vi "Climb Logic Core.vi"(11 "Climb Controls":T2) -> (3 "Climb Outputs":T1, 5 "Climbing Override":bool)   [LabVIEW 2017]
uses:
  Climb Controls.ctl
  Climb Outputs.ctl
  Robot Global Data.vi
panel:
  in  "Hook Deploy":bool
  in  "Ramp Tail":bool
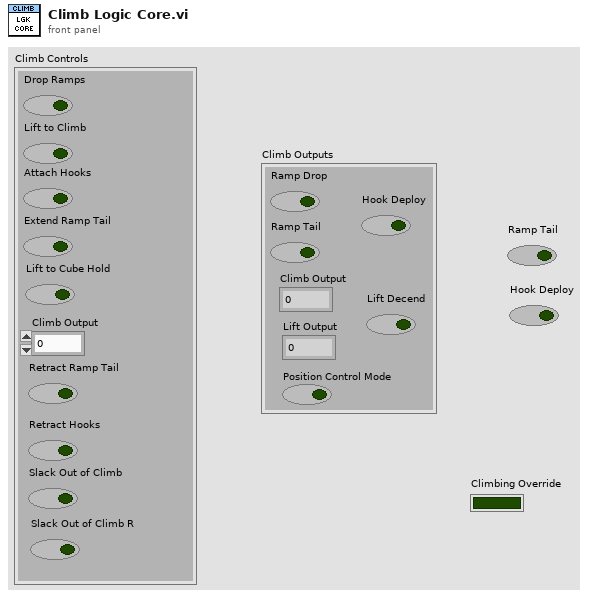
[diagram p1: front panel]
types:
  T1 = typedef "Climb Outputs.ctl" = cluster{"Ramp Drop":bool, "Ramp Tail":bool, "Climb Output":dbl, "Lift Output":dbl, "Position Control Mode":bool, "Hook Deploy":bool, "Lift Decend":bool}
  T2 = typedef "Climb Controls.ctl" = cluster{"Drop Ramps":bool, "Lift to Climb":bool, "Attach Hooks":bool, "Extend Ramp Tail":bool, "Climb Output":dbl, "Lift to Cube Hold":bool, "Retract Ramp Tail":bool, "Retract Hooks":bool, "Slack Out of Climb":bool, "Slack Out of Climb R":bool}
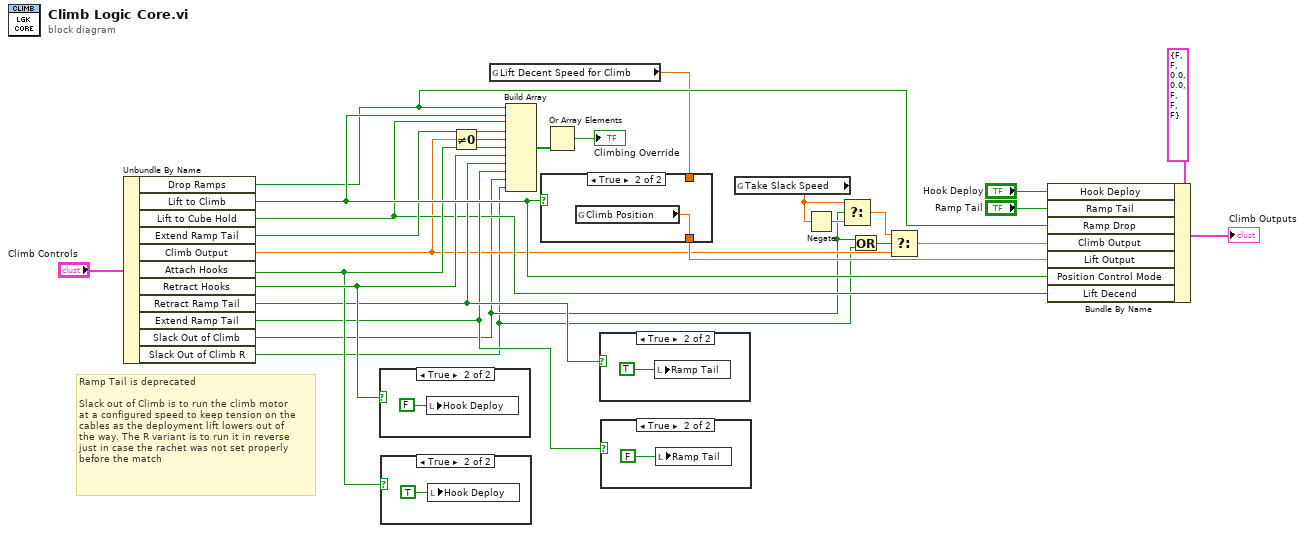
[diagram p0: block diagram]
diagram:
  # "Ramp Tail is deprecated\n\nSlack out of Climb is to run the climb motor\nat a configured speed to keep tension on the\ncables as the deployment lift lowers out of\nthe way. The R variant is to run it in reverse\njust in case the rachet was not set properly\nbefore the match"
  n1 = Unbundle By Name("Climb Controls") -> ("Drop Ramps"=w17:bool, "Lift to Climb"=w21:bool, "Lift to Cube Hold"=w9:bool, "Extend Ramp Tail"=w19:bool, "Climb Output"=w4:dbl, "Attach Hooks"=w14:bool, "Retract Hooks"=w15:bool, "Retract Ramp Tail"=w13:bool, "Extend Ramp Tail"=w12:bool, "Slack Out of Climb"=w2:bool, "Slack Out of Climb R"=w1:bool)
  n2 = case shown="True" w15 {
    frame False {
    }
    frame True {
      n3 = local write "Hook Deploy"(FALSE) -> ()
    }
  }
  n4 = case shown="True" w14 {
    frame False {
    }
    frame True {
      n5 = local write "Hook Deploy"(TRUE) -> ()
    }
  }
  n6 = Not Equal To 0?(x=w4) -> (x != 0?=w22:bool)
  n7 = global read "Robot Global Data.vi" "Lift Decent Speed for Climb"() -> (w10:dbl)
  n8 = Build Array(w17, w21, w9, w19, w22, w14, w15, w13, w12, w2, w1) -> (w24:bool[])
  n9 = case shown="True" w21 {
    tunnel: [w29 w30] -> w20
    tunnel: w10 -> [w29 _]
    frame False {
    }
    frame True {
      n10 = global read "Robot Global Data.vi" "Climb Position"() -> (w30:dbl)
    }
  }
  n11 = Or Array Elements(Boolean array=w24) -> (logical OR=→"Climbing Override":bool)
  n12 = case shown="True" w13 {
    frame False {
    }
    frame True {
      n13 = local write "Ramp Tail"(TRUE) -> ()
    }
  }
  n14 = case shown="True" w12 {
    frame False {
    }
    frame True {
      n15 = local write "Ramp Tail"(FALSE) -> ()
    }
  }
  n16 = global read "Robot Global Data.vi" "Take Slack Speed"() -> (w5:dbl)
  n17 = Negate(x=w5) -> (-x=w6:dbl)
  n18 = Select(t=w5, s=w2, f=w6) -> (s? t:f=w7:dbl)
  n19 = Or(x=w2, y=w1) -> (x .or. y?=w8:bool)
  n20 = Select(t=w7, s=w8, f=w4) -> (s? t:f=w3:dbl)
  n21 = Bundle By Name(cluster=T1 {"Ramp Drop"=FALSE, "Ramp Tail"=FALSE, "Climb Output"=0.0, "Lift Output"=0.0, "Position Control Mode"=FALSE, "Hook Deploy"=FALSE, "Lift Decend"=FALSE}, "Hook Deploy"="Hook Deploy", "Ramp Tail"="Ramp Tail", "Ramp Drop"=w17, "Climb Output"=w3, "Lift Output"=w20, "Position Control Mode"=w21, "Lift Decend"=w9) -> (→"Climb Outputs":T1)
